vi "GV PockelsScalingFactorEnable.vi"() -> ()   [LabVIEW 2017]
panel:
  out "PockelsScalingFactorEnable":bool
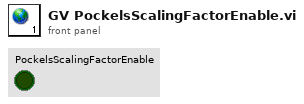
[diagram p1: front panel]
diagram:
